vi "Untitled 7.vi"   [LabVIEW 2016]
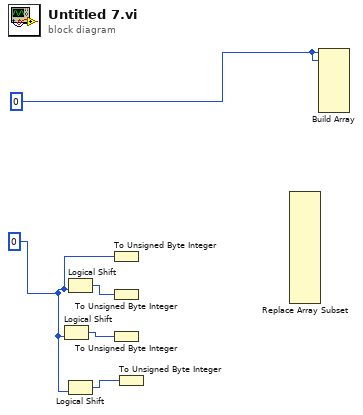
[diagram p0: block diagram]
diagram:
  w4 = u32 0
  w5 = 0
  n1 = Logical Shift(x=w4) -> (x << y=w2:u32)  [unwired: 1 in]
  n2 = Logical Shift(x=w4) -> (x << y=w1:u32)  [unwired: 1 in]
  n3 = Logical Shift(x=w4) -> (x << y=w3:u32)  [unwired: 1 in]
  n4 = To Unsigned Byte Integer(number=w4) -> ()  [unwired: 1 out]
  n5 = To Unsigned Byte Integer(number=w1) -> ()  [unwired: 1 out]
  n6 = To Unsigned Byte Integer(number=w2) -> ()  [unwired: 1 out]
  n7 = To Unsigned Byte Integer(number=w3) -> ()  [unwired: 1 out]
  n8 = Replace Array Subset() -> ()  [unwired: 13 in, 1 out]
  n9 = Build Array(w5, w5) -> ()  [unwired: 6 in, 1 out]
